vi "ListenForConnection.vi"(8 "error in (no error)":errorcluster, 9 "timeout (2000 ms)":i32=2000, 11 "Listener":refnum<class "Connection.lvclass">) -> (0 "error out":errorcluster, 1 "New connection":bool, 2 "Connection":refnum<class "Connection.lvclass">, 3 "Listener out":refnum<class "Connection.lvclass">)   [LabVIEW 2013, in "Connection_GOSPL.lvlib" / "Connection.lvclass"]
uses:
  Connection.lvclass
  Connection.lvclass/Connection.ctl
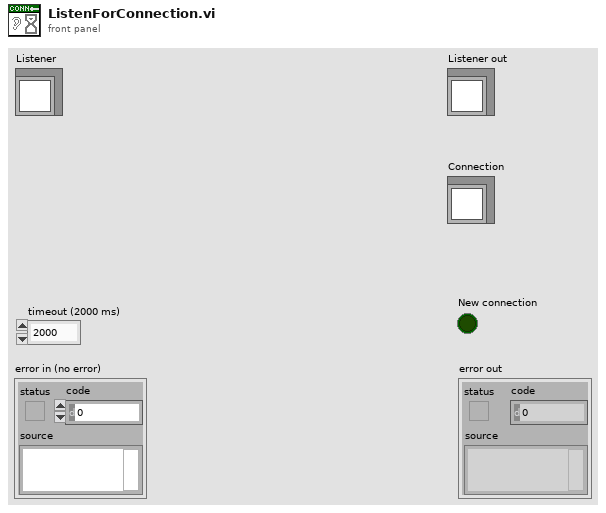
[diagram p1: front panel]
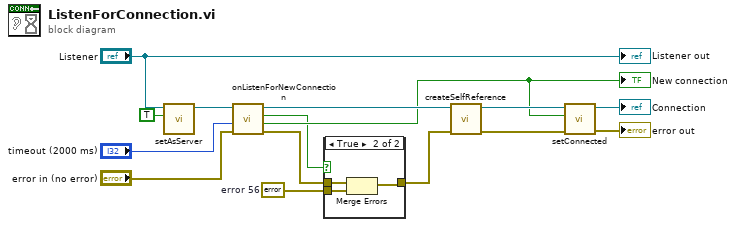
[diagram p0: block diagram]
diagram:
  w4 = errorcluster {"status"=TRUE, "code"=56, "source"="Connection_GOSPL.lvlib:Connection.lvclass:ListenForConnection.vi"}  # error 56
  n1 = call "setAsServer.vi"("server"=TRUE, "Connection in"="Listener") -> ("Connection out"=w2:refnum<class "Connection.lvclass">)  [unwired: 9 in]
  n2 = call-dynamic "onListenForNewConnection.vi"("error in (no error)"="error in (no error)", "timeout (ms)"="timeout (2000 ms)", "Listener"=w2) -> ("error out"=w7:errorcluster, "New connection"=w8:bool, "timed out"=w5:bool, "New Connection"=w11:refnum<class "Connection.lvclass">)  [unwired: 5 in]
  "New connection" <- w8
  n3 = case shown="True" w5 {
    tunnel: w4 -> [_ w19]
    tunnel: w7 -> [w16 w18]
    tunnel: [w16 w17] -> w6
    frame False {
    }
    frame True {
      n4 = Merge Errors(w18, w19) -> (w17:errorcluster)
    }
  }
  n5 = call "createSelfReference.vi"("error in (no error)"=w6, "Connection in"=w11) -> ("error out"=w9:errorcluster, "Connection out"=w10:refnum<class "Connection.lvclass">)  [unwired: 8 in]
  n6 = call "setConnected.vi"("error in (no error)"=w9, "connected"=w8, "Connection in"=w10) -> ("error out"=→"error out":errorcluster, "Connection out"=→"Connection":refnum<class "Connection.lvclass">)  [unwired: 7 in]
  "Listener out" <- "Listener"
